vi "mlink_pwm_init.vi"(4 "channel B duty":sgl, 6 "channel A duty":sgl, 7 "PWM module":enum8{"None", "PWM1", "PWM2", "PWM3"}(ring)=enum."PWM1", 8 "error in (no error)":errorcluster, 9 "period":u32=1000 min=2 max=500000, 10 "active LOW":u8, 11 "connection ID":i32=-1) -> (0 "error out":errorcluster, 3 "connection ID out":i32)   [LabVIEW 2009, in "MicroDAQ.lvlib" / "mlink.lvlib"]
doc: "This function initializes MicroDAQ PWM module. Each PWM module has A and B channel which can generate PWM waveform with different duty and same period defined for PWM module. PWM waveform period is defined in microseconds (us) (2-500000). The function allows to \ngenerate inverted PWM waveform by setting active_low variable to 1. The duty_a and duty_b determines initial PWM duty (0-100)."
uses:
  <instrlib>/MicroDAQ/Mlink library wraper/mlink.lvlib
  <instrlib>/MicroDAQ/MLink32.dll
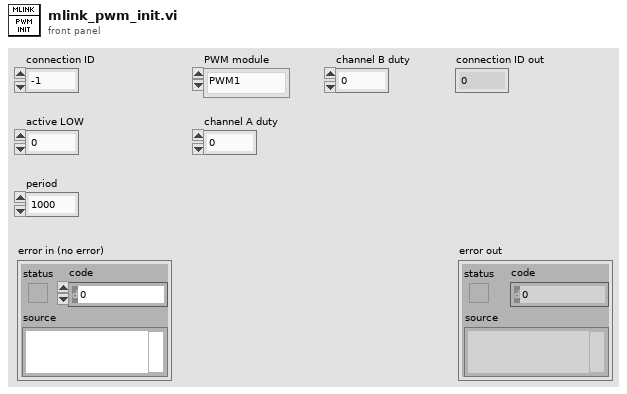
[diagram p1: front panel]
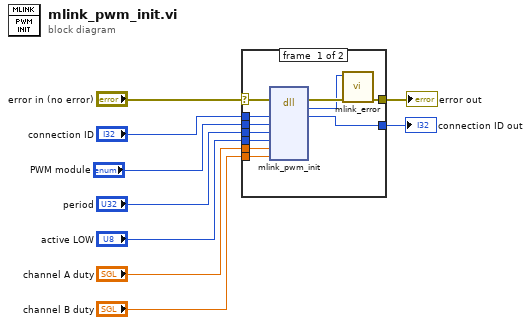
[diagram p0: block diagram]
diagram:
  n1 = case shown="No Error" "error in (no error)" {
    selector: "error in (no error)" -> [w15 w22]
    tunnel: "connection ID" -> [w20 w21]
    tunnel: [w19 w21] -> w8
    tunnel: "period" -> [w18 _]
    tunnel: "channel A duty" -> [w17 _]
    tunnel: "channel B duty" -> [w16 _]
    tunnel: "PWM module" -> [w14 _]
    tunnel: "active LOW" -> [w13 _]
    tunnel: [w10 w22] -> w2
    frame #0 {
      n2 = dll-call lib="C:/Program Files (x86)/National Instruments/LabVIEW 2009/instr.lib/MicroDAQ/MLink32.dll" fn="mlink_pwm_init"(error in=w15, "connection ID"=w20, "module"=w14, "period"=w18, "active LOW"=w13, "channel A"=w17, "channel B"=w16) -> (error out=w12:errorcluster, "return type"=w11:i32, "connection ID"=w19:i32)  [unwired: 7 in, 1 out]
      n3 = call <instrlib>:"mlink_error.vi"("error in (no error)"=w12, "error code"=w11) -> ("error out"=w10:errorcluster)  [unwired: 9 in]
    }
    frame #1 {
    }
  }
  "connection ID out" <- w8
  "error out" <- w2
